vi "DIO Write.vi"(7 "DIO line":T1=1300 items=["FPGA LED"=6000, "Port3/DIO0"=1300, "Port3/DIO1"=1301, "Port3/DIO2"=1302, "Port3/DIO3"=1303, "Port3/DIO4"=1304, "Port3/DIO5"=1305, "Port3/DIO6"=1306, "Port3/DIO7"=1307, "Port3/DIO8"=1308, "Port3/DIO9"=1309], 8 "error in (no error)":errorcluster, 10 "data":bool, 11 "direct IO in":refnum<class "NI_Robotics_Starter Kit Direct IO_FPGA.lvclass">) -> (0 "error out":errorcluster, 3 "direct IO out":refnum<class "NI_Robotics_Starter Kit Direct IO_FPGA.lvclass">)   [LabVIEW 2017, in "NI_Robotics_Starter Kit Direct IO_FPGA.lvclass"]
uses:
  <vilib>/robotics/Starter Kit/FPGA Direct IO/NI_Robotics_Starter Kit Direct IO_FPGA.lvclass
  <vilib>/robotics/Starter Kit/Direct IO/DIO Lines.ctl
  <vilib>/robotics/Starter Kit/FPGA Direct IO/NI_Robotics_Starter Kit Direct IO_FPGA.lvclass/NI_Robotics_Starter Kit Direct IO_FPGA.ctl
  <vilib>/rvi/errors/niLvFpgaAdjustHostInterfaceError.vi
  <vilib>/Utility/error.llb/Error Cluster From Error Code.vi
  <vilib>/robotics/Starter Kit/FPGA Direct IO/Direct IO FPGA Ref.ctl
  <vilib>/rvi/interface/nirviReadWriteControl/nirviReadWriteControl.xnode
  NiFpgaLv.dll
  <vilib>/rvi/interface/Simulation/niFpgaSimulationCallBeginRW.vi
  <vilib>/robotics/Starter Kit/Direct IO/NI_Robotics_Starter Kit Direct IO.lvclass
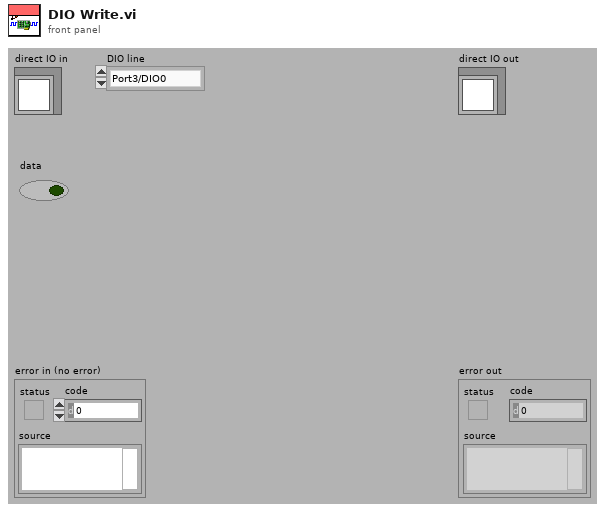
[diagram p1: front panel]
types:
  T1 = typedef "NI_Robotics_Starter Kit Direct IO.lvclass/DIO Lines.ctl" = u16
  T2 = typedef "NI_Robotics_Starter Kit Direct IO_FPGA.lvclass/Direct IO FPGA Ref.ctl" = refnum<k20>
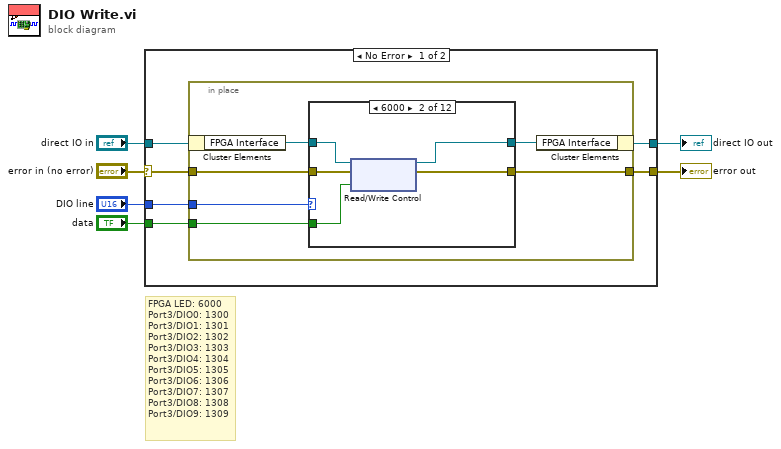
[diagram p0: block diagram]
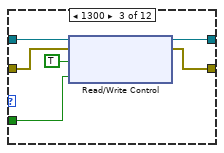
[diagram p3: hidden frame]
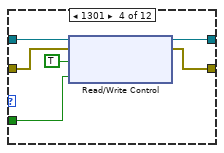
[diagram p4: hidden frame]
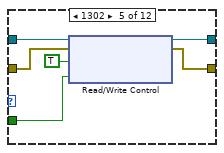
[diagram p5: hidden frame]
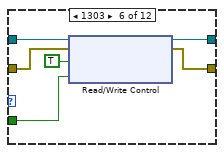
[diagram p6: hidden frame]
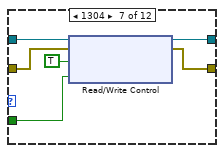
[diagram p7: hidden frame]
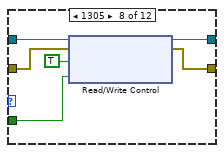
[diagram p8: hidden frame]
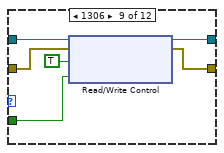
[diagram p9: hidden frame]
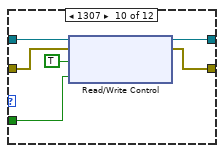
[diagram p10: hidden frame]
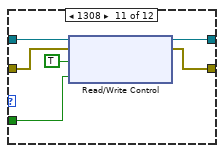
[diagram p11: hidden frame]
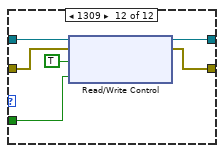
[diagram p12: hidden frame]
diagram:
  # "FPGA LED: 6000\nPort3/DIO0: 1300\nPort3/DIO1: 1301\nPort3/DIO2: 1302\nPort3/DIO3: 1303\nPort3/DIO4: 1304\nPort3/DIO5: 1305\nPort3/DIO6: 1306\nPort3/DIO7: 1307\nPort3/DIO8: 1308\nPort3/DIO9: 1309"
  n1 = case shown="No Error" "error in (no error)" {
    selector: "error in (no error)" -> [w10 w87]
    tunnel: [w9 w87] -> w2
    tunnel: "direct IO in" -> [w12 w86]
    tunnel: [w8 w86] -> w3
    tunnel: "DIO line" -> [w11 _]
    tunnel: "data" -> [w7 _]
    frame No Error {
      n2 = in-place {
        in-place-border: w11 -> [w18]
        in-place-border: w10 -> [w16]
        in-place-border: [w14] -> w9
        in-place-border: w7 -> [w13]
        n3 = in-place-cluster #1(w12) -> ("FPGA Interface"=w17:T2)
        n4 = case shown="6000" w18 {
          tunnel: w17 -> [w20 w25 w31 w37 w43 w49 w55 w61 w67 w73 w79 w85]
          tunnel: w16 -> [w19 w24 w29 w35 w41 w47 w53 w59 w65 w71 w77 w83]
          tunnel: [w20 w21 w28 w34 w40 w46 w52 w58 w64 w70 w76 w82] -> w15
          tunnel: [w19 w22 w27 w33 w39 w45 w51 w57 w63 w69 w75 w81] -> w14
          tunnel: w13 -> [_ w23 w26 w32 w38 w44 w50 w56 w62 w68 w74 w80]
          frame Default {
          }
          frame 6000 {
            n5 = xnode "Read/Write Control"("FPGA VI Reference In"=w25, "error in"=w24, "FPGA LED"=w23) -> ("FPGA VI Reference Out"=w21:T2, "error out"=w22:errorcluster)
          }
          frame 1300 {
            n6 = xnode "Read/Write Control"("FPGA VI Reference In"=w31, "error in"=w29, "Port3/DIO0_write"=TRUE ("DIO_0_write"), "Port3/DIO0"=w26) -> ("FPGA VI Reference Out"=w28:T2, "error out"=w27:errorcluster)
          }
          frame 1301 {
            n7 = xnode "Read/Write Control"("FPGA VI Reference In"=w37, "error in"=w35, "Port3/DIO1_write"=TRUE ("DIO_0_write"), "Port3/DIO1"=w32) -> ("FPGA VI Reference Out"=w34:T2, "error out"=w33:errorcluster)
          }
          frame 1302 {
            n8 = xnode "Read/Write Control"("FPGA VI Reference In"=w43, "error in"=w41, "Port3/DIO2_write"=TRUE ("DIO_0_write"), "Port3/DIO2"=w38) -> ("FPGA VI Reference Out"=w40:T2, "error out"=w39:errorcluster)
          }
          frame 1303 {
            n9 = xnode "Read/Write Control"("FPGA VI Reference In"=w49, "error in"=w47, "Port3/DIO3_write"=TRUE ("DIO_0_write"), "Port3/DIO3"=w44) -> ("FPGA VI Reference Out"=w46:T2, "error out"=w45:errorcluster)
          }
          frame 1304 {
            n10 = xnode "Read/Write Control"("FPGA VI Reference In"=w55, "error in"=w53, "Port3/DIO4_write"=TRUE ("DIO_0_write"), "Port3/DIO4"=w50) -> ("FPGA VI Reference Out"=w52:T2, "error out"=w51:errorcluster)
          }
          frame 1305 {
            n11 = xnode "Read/Write Control"("FPGA VI Reference In"=w61, "error in"=w59, "Port3/DIO5_write"=TRUE ("DIO_0_write"), "Port3/DIO5"=w56) -> ("FPGA VI Reference Out"=w58:T2, "error out"=w57:errorcluster)
          }
          frame 1306 {
            n12 = xnode "Read/Write Control"("FPGA VI Reference In"=w67, "error in"=w65, "Port3/DIO6_write"=TRUE ("DIO_0_write"), "Port3/DIO6"=w62) -> ("FPGA VI Reference Out"=w64:T2, "error out"=w63:errorcluster)
          }
          frame 1307 {
            n13 = xnode "Read/Write Control"("FPGA VI Reference In"=w73, "error in"=w71, "Port3/DIO7_write"=TRUE ("DIO_0_write"), "Port3/DIO7"=w68) -> ("FPGA VI Reference Out"=w70:T2, "error out"=w69:errorcluster)
          }
          frame 1308 {
            n14 = xnode "Read/Write Control"("FPGA VI Reference In"=w79, "error in"=w77, "Port3/DIO8_write"=TRUE ("DIO_0_write"), "Port3/DIO8"=w74) -> ("FPGA VI Reference Out"=w76:T2, "error out"=w75:errorcluster)
          }
          frame 1309 {
            n15 = xnode "Read/Write Control"("FPGA VI Reference In"=w85, "error in"=w83, "Port3/DIO9_write"=TRUE ("DIO_0_write"), "Port3/DIO9"=w80) -> ("FPGA VI Reference Out"=w82:T2, "error out"=w81:errorcluster)
          }
        }
        n16 = in-place-cluster #1("FPGA Interface"=w15) -> (w8:refnum<class "NI_Robotics_Starter Kit Direct IO_FPGA.lvclass">)
      }
    }
    frame Error {
    }
  }
  "error out" <- w2
  "direct IO out" <- w3
